vi "s-lab第8章 节点1-5.vi"() -> ()   [LabVIEW 2013]
panel:
  out "数值显示":dbl
  in  "数值输入":dbl
  in  "数值条件":dbl
  out "布尔 2":bool
  in  "布尔":bool
  out "y=3*x+100":dbl
  in  "x3":dbl
  in  "停止":bool
  out "数值 2":dbl
  in  "数值":dbl
  out "Y=10*X+100":dbl
  in  "X":dbl
  # "例 1"
  # "例 2"
  # "例 3"
  # "例 4"
  # "例 5"
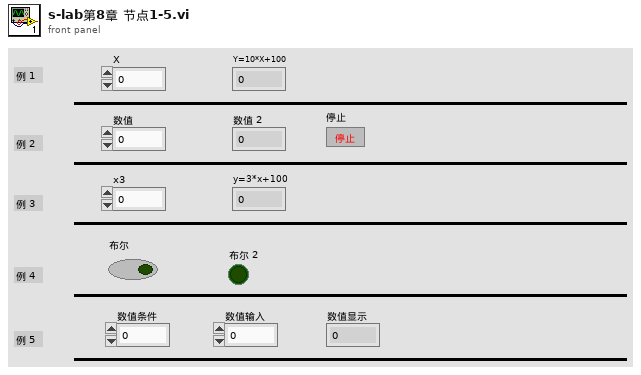
[diagram p1: front panel]
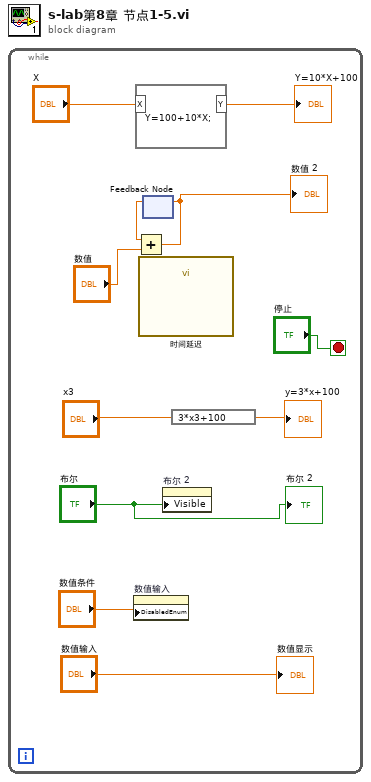
[diagram p0: block diagram]
diagram:
  n1 = while {
    stop <- "停止" stop-if-true
    n2 = property on="数值输入" class="DigNum (严格)"("DisabledEnum"="数值条件") -> ()  [unwired: 2 in, 2 out]
    n3 = formula code="Y=100+10*X;"("X"="X") -> ("Y"=→"Y=10*X+100":dbl)
    n4 = call "时间延迟"() -> ()  [unwired: 11 in, 1 out]
    n5 = feedback #1() -> (w9:dbl)  [unwired: 1 in]
    n6 = Add(x=w9, y="数值") -> (x+y=w8:dbl)
    "数值 2" <- w8
    n7 = feedback-in #1(w8) -> ()
    n8 = property on="布尔 2" class="Bool (严格)"("Visible"="布尔") -> ()  [unwired: 2 in, 2 out]
    n9 = expression code="3*x3+100"("x3") -> (→"y=3*x+100":dbl)
    "布尔 2" <- "布尔"
    "数值显示" <- "数值输入"
  }
